vi "UI Event Handler.vi"() -> ()   [LabVIEW 2018]
uses:
  <vilib>/Utility/miscctls.llb/LVPoint32TypeDef.ctl
panel:
  out "Coords":T1
  out "current time":timestamp
  in  "Time Check":bool
  out "Iteration":i32
  in  "Stop":bool
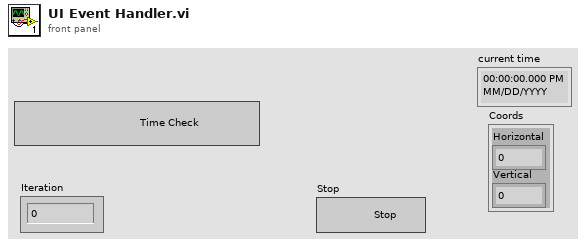
[diagram p1: front panel]
types:
  T1 = typedef "LVPoint32TypeDef.ctl" = cluster{"Horizontal":i32, "Vertical":i32}
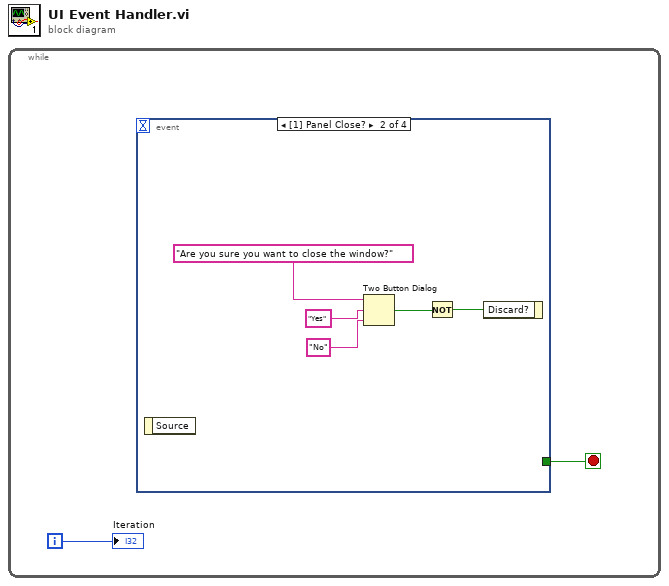
[diagram p0: block diagram]
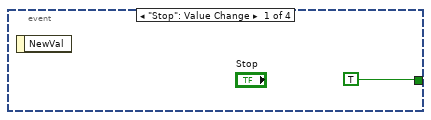
[diagram p2: hidden frame]
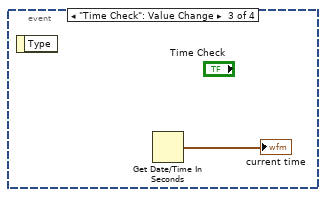
[diagram p3: hidden frame]
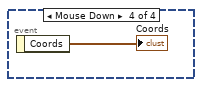
[diagram p4: hidden frame]
diagram:
  n1 = while {
    i -> [w2]
    stop <- w1 stop-if-true
    n2 = event shown="[1] Panel Close?" {
      selector: _ -> [_ _ _ _]
      dyn-events: _ -> [_ _ _ _]
      timeout: _ -> [_ _ _ _]
      tunnel: [TRUE _ _ _] -> w1
      event "Stop": Value Change {
        n3 = event-data() -> ()  [unwired: 1 in, 1 out]
      }
      event Panel Close? {
        n4 = event-data() -> ()  [unwired: 1 in, 1 out]
        n5 = Two Button Dialog(message="Are you sure you want to close the window?", 1:"No", 2:"Yes") -> (T button?=w7:bool)
        n6 = Not(x=w7) -> (.not. x?=w8:bool)
        n7 = event-data("Discard?"=w8) -> ()  [unwired: 1 in, 1 out]
      }
      event "Time Check": Value Change {
        n8 = event-data() -> ()  [unwired: 1 in, 1 out]
        n9 = Get Date/Time In Seconds() -> (seconds since 1Jan1904=→"current time":timestamp)
      }
      event Mouse Down {
        n10 = event-data() -> ("Coords"=→"Coords":T1)  [unwired: 1 in]
      }
    }
    "Iteration" <- w2
  }
